vi "Set DDG Times.vi"(8 "error in (no error)":errorcluster, 9 "t2":dbl, 10 "t1":dbl, 11 "t0":dbl) -> (0 "error out":errorcluster, 3 "function return":u32)   [LabVIEW 2014, in "atmcd32d.lvlib"]
doc: "unsigned int WINAPI SetDDGTimes(double t0, double t1, double t2);"
uses:
  atmcd32d.lvlib
  atmcd32d.dll
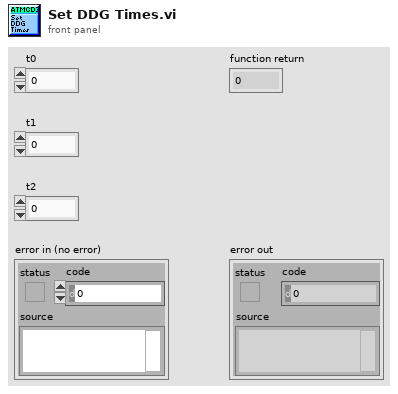
[diagram p1: front panel]
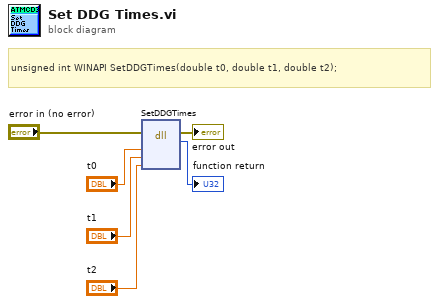
[diagram p0: block diagram]
diagram:
  # "unsigned int WINAPI SetDDGTimes(double t0, double t1, double t2);"
  n1 = dll-call lib="C:/Users/Bakir/Documents/Lambda2-Testing/lib/Andorlib/atmcd32d.*" fn="SetDDGTimes"(error in="error in (no error)", "t0"="t0", "t1"="t1", "t2"="t2") -> (error out=→"error out":errorcluster, →"function return":u32)  [unwired: 5 in, 1 out]
